vi "class_data.vi"() -> ()   [LabVIEW 2010, in "GenericScanHead.lvclass"]
uses:
  GenericScanHead.lvclass
panel:
  in  "latest instance":refnum<class "GenericScanHead.lvclass">
  in  "trajectory queue name":string="trajectory queue"
  in  "offset queue name":string="scan head offset queue"
  in  "locked by":string="DL090202ScanHead.lvclass:run.vi > GenericScanHead.lvclass:manager.vi > main.vi"
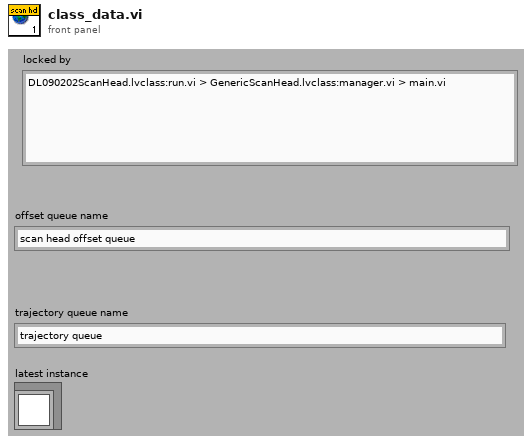
[diagram p1: front panel]
diagram:
